vi "H5PTcreate_fl.vi"(4 "compression":i32, 5 "dset_name":string, 6 "chunk_size":i64, 7 "dtype_id":i32, 8 "error in (no error)":errorcluster, 11 "loc_id":i32) -> (0 "error out":errorcluster, 3 "table_id":i32)   [LabVIEW 2009]
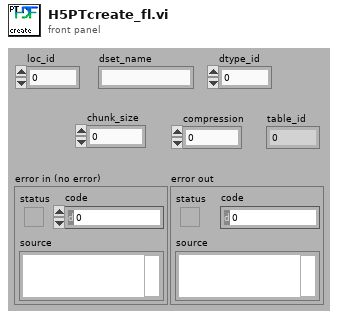
[diagram p1: front panel]
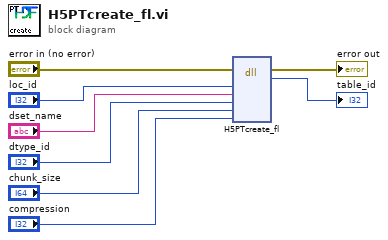
[diagram p0: block diagram]
diagram:
  n1 = dll-call lib="hdf5_hldll" fn="H5PTcreate_fl"(error in="error in (no error)", "loc_id"="loc_id", "dset_name"="dset_name", "dtype_id"="dtype_id", "chunk_size"="chunk_size", "compression"="compression") -> (error out=→"error out":errorcluster, "return type"=→"table_id":i32)  [unwired: 7 in, 1 out]
